vi "TAFTraceWindow_AddSubscriber.vi"(8 "ErrorIn":errorcluster, 10 "CmdData":variant, 11 "TAFTraceWindow in":refnum<class>) -> (0 "ErrorOut":errorcluster, 2 "ReplyData":variant, 3 "TAFTraceWindow out":refnum<class>, 4 "Exit":bool)   [LabVIEW 2021, in "TAFTraceWindow.lvclass"]
uses:
  TAFTraceWindow.lvclass
  TAFTraceWindow.lvclass/TAFTraceWindow.ctl
  FilterFunction.ctl
  FilterConfiguration.ctl
  FilterSubscriberConfiguration.ctl
  4471e090-8e64-498f-a1be-083322230ba5.vi
  C:/Localdata/Projects/TriekselSoft/TriekselsoftApplicationFramework/Source/.Externals/Library_TAF/YAFTAF/YAFTAF.lvclass
  C:/Localdata/Projects/TriekselSoft/TriekselsoftApplicationFramework/Source/.Externals/Library_TAF/YActor/YActor.lvclass
  C:/Localdata/Projects/TriekselSoft/TriekselsoftApplicationFramework/Source/.Externals/Interface_UserInterface_IFrontPanel/IFrontPanel/IFrontPanel.lvclass
  C:/Localdata/Projects/TriekselSoft/TriekselsoftApplicationFramework/Source/.Externals/Interface_TAF_IInterface/IInterface/IInterface.lvclass
  C:/Localdata/Projects/TriekselSoft/TriekselsoftApplicationFramework/Source/.Externals/Interface_Object_ICreateDestroy/ICreateDestroy/ICreateDestroy.lvclass
  C:/Localdata/Projects/TriekselSoft/TriekselsoftApplicationFramework/Source/.Externals/Interface_Object_IPersistentData/IPersistentData/IPersistentData.lvclass
  C:/Localdata/Projects/TriekselSoft/TriekselsoftApplicationFramework/Source/.Externals/Interface_TAF_ITAFObject/ITAFObject/ITAFObject.lvclass
  C:/Localdata/Projects/TriekselSoft/TriekselsoftApplicationFramework/Source/.Externals/Library_TAF_TraceWindow/TAFTraceWindow/TAFTraceWindow.lvclass
  C:/Localdata/Projects/TriekselSoft/TriekselsoftApplicationFramework/Source/.Externals/Interface_TAF_TraceSubscriptor/ITAFFilteredTrace/ITAFFilteredTrace.lvclass
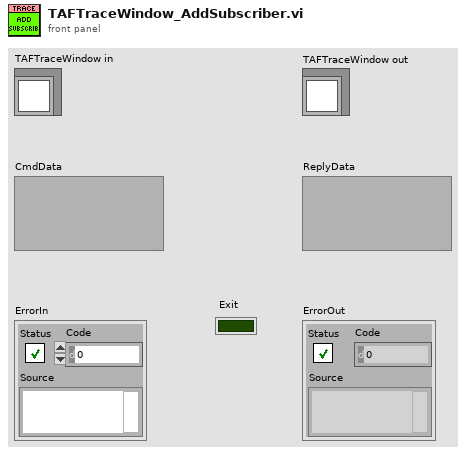
[diagram p1: front panel]
types:
  T1 = typedef "TAFTraceWindow.lvclass/FilterConfiguration.ctl" = cluster{"TraceColumn":i32, "FilterFunction":T2, "SearchText":string}
  T2 = typedef "TAFTraceWindow.lvclass/FilterFunction.ctl" = enum16{"Exact", "Regex"}
  T3 = typedef "TAFTraceWindow.lvclass/FilterSubscriberConfiguration.ctl" = cluster{"Name":string, "TargetQueue":refnum<queue>, "Configs":T1[]}
  T4 = cluster{"Name":string, "TargetQueue":refnum<queue>, "Configs":T1[]}[]
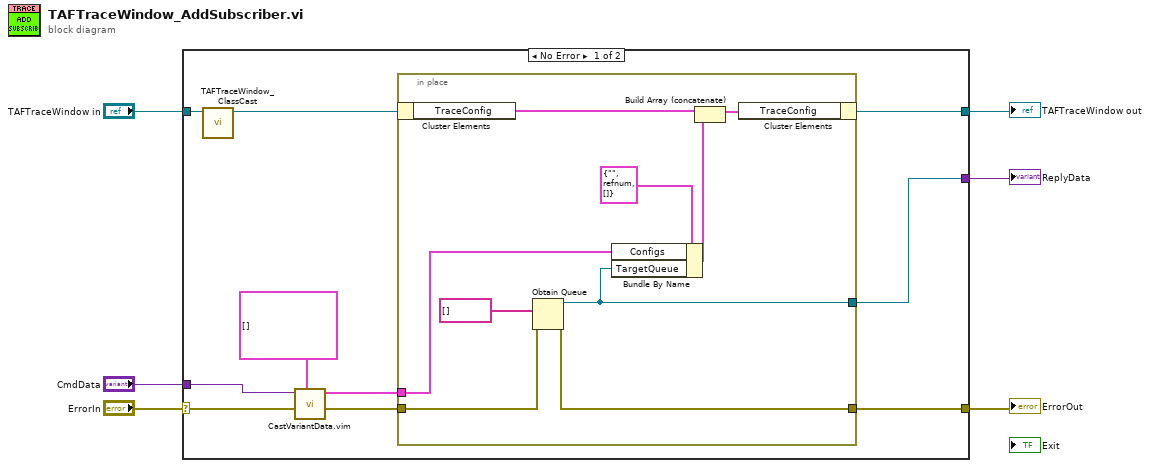
[diagram p0: block diagram]
diagram:
  n1 = case shown="No Error" "ErrorIn" {
    selector: "ErrorIn" -> [w16 w28]
    tunnel: [w9 w28] -> w5
    tunnel: [w8 w27] -> w3
    tunnel: "CmdData" -> [w14 w27]
    tunnel: "TAFTraceWindow in" -> [w15 w26]
    tunnel: [w7 w26] -> w1
    frame No Error {
      n2 = call "TAFTraceWindow_ClassCast.vi"("TAFTraceWindow in"=w15) -> ("TAFTraceWindow out"=w12:refnum<class "TAFTraceWindow.lvclass">)  [unwired: 10 in]
      n3 = call "CastVariantData.vim"("Type"=T1[] [] ("Filters"), "ErrorIn"=w16, "DataIn"=w14) -> ("ErrorOut"=w10:errorcluster, "DataOut"=w11:T1[])  [unwired: 7 in]
      n4 = in-place {
        in-place-border: w11 -> [w22]
        in-place-border: w10 -> [w18]
        in-place-border: [w19] -> w9
        in-place-border: [w17] -> w8
        n5 = in-place-cluster #1(w12) -> ("TraceConfig"=w25:T4)
        n6 = Obtain Queue(element data type=string[] [], error in (no error)=w18) -> (queue out=w17:refnum<queue>, error out=w19:errorcluster)  [unwired: 3 in, 1 out]
        n7 = Bundle By Name(cluster=T3 {"Name"="", "TargetQueue"=refnum, "Configs"=[]} ("FilterSubscriberConfiguration"), "Configs"=w22, "TargetQueue"=w17) -> (w21:T3)
        n8 = Build Array (concatenate)(w25, w21) -> (w20:T3[])
        n9 = in-place-cluster #1("TraceConfig"=w20) -> (w7:refnum<class "TAFTraceWindow.lvclass">)
      }
    }
    frame Error {
    }
  }
  "ErrorOut" <- w5
  "TAFTraceWindow out" <- w1
  "ReplyData" <- w3
